vi "Unregister XNET Database.vi"(8 "error in (no error)":errorcluster, 11 "alias":string) -> (0 "error out":errorcluster)   [LabVIEW 2017]
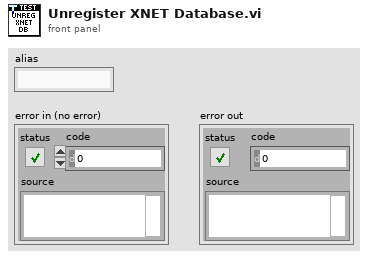
[diagram p1: front panel]
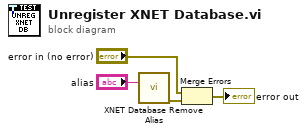
[diagram p0: block diagram]
diagram:
  n1 = call <vilib>:"XNET Database Remove Alias.vi"("alias"="alias") -> ("error out"=w3:errorcluster)  [unwired: 14 in]
  n2 = Merge Errors("error in (no error)", w3) -> (→"error out":errorcluster)
